vi "Get Parent Node ID from ID.vi"(8 "error in (no error)":errorcluster, 11 "Node ID":string) -> (0 "error out":errorcluster, 3 "Parent ID":string)   [LabVIEW 2015, in "Configuration Tool.lvlib"]
uses:
  Configuration Tool.lvlib
  <vilib>/NI/Configuration Framework/Node/NISE_CEF_Node.lvclass/NISE_CEF_Node.ctl
  <vilib>/NI/Configuration Framework/Node/ReadParent.vi
  <vilib>/NI/Configuration Framework/Node/NISE_CEF_Node.lvclass
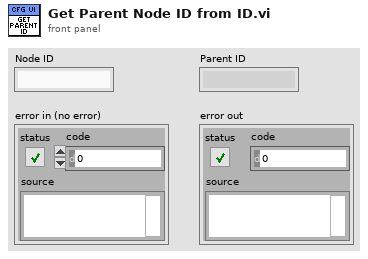
[diagram p1: front panel]
types:
  T1 = typedef "NISE_CEF_Node.lvclass/NodeRef.ctl" = refnum<data-value>
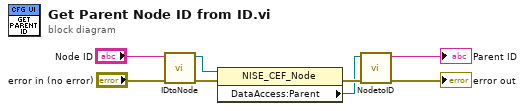
[diagram p0: block diagram]
diagram:
  n1 = call <vilib>:"IDtoNode.vi"("error in"="error in (no error)", "ID"="Node ID") -> ("error out"=w7:errorcluster, "node ref"=w4:T1)  [unwired: 7 in, 1 out]
  n2 = property on="Property Node" class="NISE_CEF_Node"(reference=w4, error in=w7) -> (error out=w5:errorcluster, "DataAccess:Parent"=w2:T1)  [unwired: 1 out]
  n3 = call <vilib>:"NodetoID.vi"("error in"=w5, "node ref"=w2) -> ("error out"=→"error out":errorcluster, "ID"=→"Parent ID":string)  [unwired: 8 in]
